vi "Main.vi"() -> ()   [LabVIEW 2012]
uses:
  UIAction.ctl
  UIActionQueueElement.ctl
  HeaterAction.ctl
  HeaterActionQueueElement.ctl
  MFCAction.ctl
  MFCActionQueueElement.ctl
  libs/LV-Utilities/LV-Utilities.lvlib
  LogAction.ctl
  LogActionQueueElement.ctl
  <vilib>/Utility/error.llb/DialogType.ctl
  HardwareAction.ctl
  HardwareActionQueueElement.ctl
  HeaterConfigurationGlobalAction.ctl
  MFCConfigurationGlobalAction.ctl
panel:
  in  "Chamber":u16(ring) items=["Chamber Name"]
  in  "NEXT CHAMBER":bool
  in  "PREVIOUS CHAMBER":bool
  in  "REMOVE CHAMBER":bool
  in  "ADD CHAMBER":bool
  out "MFC COM Port":u8=1
  out "Heater COM Port":u8=1
  in  "CONFIGURE HEATER":bool
  in  "PLOT MFC":bool
  in  "PLOT HEATER":bool
  in  "LOG START":bool
  out "Log Running?":bool
  in  "RESET":bool
  in  "SAVE":bool
  in  "OPEN":bool
  out "MFC Serial Number":string="Serial Number"
  in  "SELECT CONFIG":bool
  out "Setup File":path
  in  "CONFIGURE MFC":bool
  out "Heater Actual Slide":dbl(slide) scale=0.0..200.0 scale format="%#.1f"
  out "Heater Actual (C)":dbl=nan format="%.1f"
  out "Heater Setpoint Slide":dbl(slide) scale=0.0..200.0 scale format="%#.1f"
  out "Heater Setpoint (C)":dbl=nan format="%.1f"
  out "Heater State":enum16{"Not Connected", "Run", "Standby"}(ring)
  out "MFC Actual Slide":dbl(slide) scale=0.0..1000.0 scale format="%#.1f"
  out "MFC Actual (mL/min)":dbl=nan format="%.1f"
  out "MFC Setpoint Slide":dbl(slide) scale=0.0..1000.0 scale format="%#.1f"
  out "MFC Setpoint (mL/min)":dbl=nan format="%.1f"
  out "MFC Valve State":T1(ring)
  in  "DONE":bool
  # "Vacuum Pump"
  # "COM Port:"
  # "COM Port:"
  # "LOG"
  # "SETUP"
  # "Config File:"
  # "Actual"
  # "Setpoint"
  # "Actual"
  # "Setpoint"
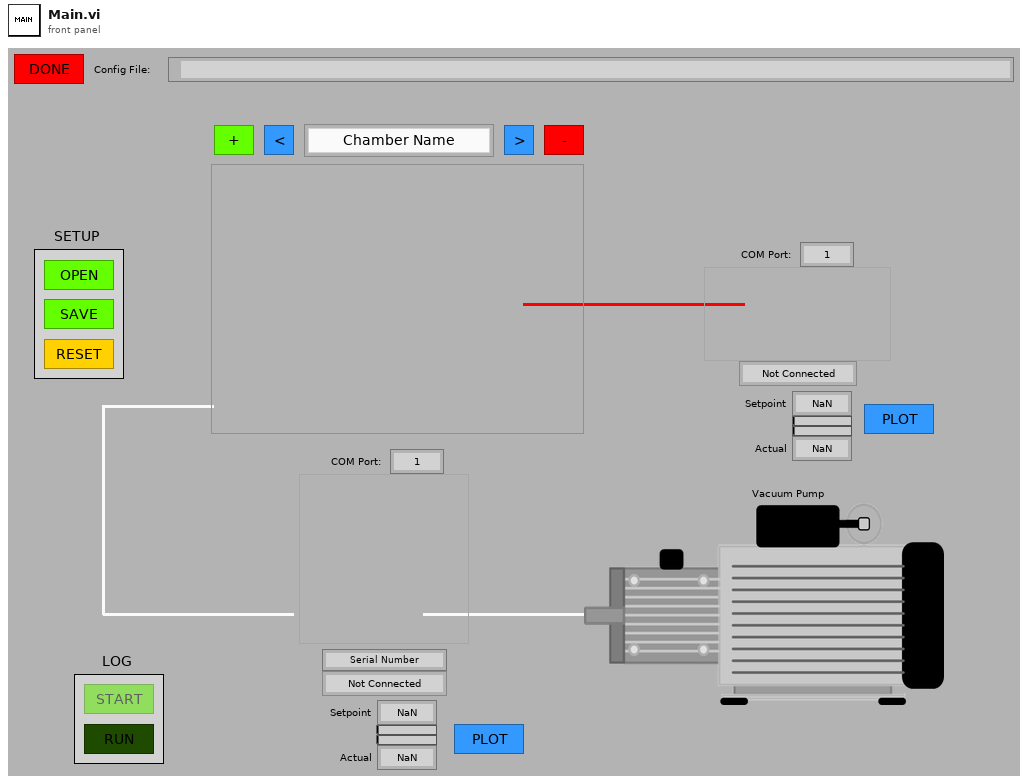
[diagram p1: front panel]
types:
  T1 = enum16{"Not Connected", "Automatic", "Closed", "Purge"}
  T2 = typedef "DataStructures.ctl" = cluster{"Display":refnum<notifier>, "Log":refnum<queue>}
  T3 = typedef "ActionQueues.ctl" = cluster{"UI Action":refnum<queue>, "Hardware Action":refnum<queue>, "Heater Action":refnum<queue>, "MFC Action":refnum<queue>, "Log Action":refnum<queue>}
  T4 = typedef "ExecutableConfiguration.ctl" = cluster{"Default Chamber Folder Path":path, "Default Log Folder Path":path, "Default Monitor":i32, "Center on Monitor?":bool}
  T5 = typedef "MFCActionQueueElement.ctl" = cluster{"Action":T6, "Data":variant}
  T6 = typedef "MFCAction.ctl" = enum16{"Initialize", "Start", "Read", "Write", "Stop", "Error", "Shutdown"}
  T7 = typedef "HeaterActionQueueElement.ctl" = cluster{"Action":T8, "Data":variant}
  T8 = typedef "HeaterAction.ctl" = enum16{"Initialize", "Start", "Read", "Write", "Stop", "Error", "Shutdown"}
  T9 = typedef "HardwareActionQueueElement.ctl" = cluster{"Action":T10, "Data":variant}
  T10 = typedef "HardwareAction.ctl" = enum16{"Initialize", "Collect", "Shutdown"}
  T11 = typedef "LogActionQueueElement.ctl" = cluster{"Action":T12, "Data":variant}
  T12 = typedef "LogAction.ctl" = enum16{"Initialize", "Start", "Log", "Stop", "Error", "Shutdown"}
  T13 = typedef "MFCConfigurationGlobalAction.ctl" = enum16{"Init", "Get", "Set", "Add", "Remove", "Reset"}
  T14 = typedef "HeaterConfigurationGlobalAction.ctl" = enum16{"Init", "Get", "Set", "Add", "Remove", "Reset"}
  T15 = enum8{"Enabled", "Disabled", "Disabled and Grayed Out"}
  T16 = typedef "UIActionQueueElement.ctl" = cluster{"Action":T17, "Data":variant}
  T17 = typedef "UIAction.ctl" = enum16{"Initialize", "Connect", "MFC Connected", "Heater Connected", "Disconnect", "MFC Disconnected", "Heater Disconnected", "Configure MFC", "Configure Heater", "Open Log", "Close Log", "Shutdown"}
  T18 = typedef "Setup.ctl" = cluster{"Chamber Name":string, "Log Folder Path":path, "Heater":T19, "MFC":T20}
  T19 = typedef "HeaterConfiguration.ctl" = cluster{"COM Port":u8, "Setpoint":dbl, "Standby?":bool}
  T20 = typedef "MFCConfiguration.ctl" = cluster{"COM Port":u32, "Timeout (msec)":u32, "Setpoint":dbl, "Valve State":T21, "Gas":T22, "Units":T23, "Serial Number":string, "Firmware Version":string}
  T21 = typedef "Sierra-M100.lvlib/ValveState.ctl" = enum16{"Automatic", "Closed", "Purge"}
  T22 = typedef "Sierra-M100.lvlib/Gas.ctl" = enum16{"Air", "Argon", "CO2", "CO", "Helium", "Hydrogen", "Methane", "Nitrogen", "Nitrous Oxide", "Oxygen"}
  T23 = typedef "Sierra-M100.lvlib/Units.ctl" = enum16{"scc/s", "scc/m", "scc/H", "Ncc/s", "Ncc/m", "Ncc/H", "SCF/s", "SCF/m", "SCF/H", "NM3/s", "NM3/m", "NM3/H", "SM3/s", "SM3/m", "SM3/H", "sl/s", "sl/m", "sl/H", "NL/s", "NL/m", "Nl/H", "g/s", "g/m", "g/H", "kg/s", "kg/m", "kg/H", "lb/s", "lb/m", "lb/H"}
  T24 = cluster{"Setpoint (mL/min)":dbl, "Actual (mL/min)":dbl}[]
  T25 = cluster{"Setpoint (mL/min)":dbl, "Actual (mL/min)":dbl}
  T26 = typedef "DialogType.ctl" = u16
  T27 = typedef "HardwareDisplayData.ctl" = cluster{"Heater":dbl, "MFC":dbl}
  T28 = typedef "MFCDisplayValveState.ctl" = enum16{"Not Connected", "Automatic", "Closed", "Purge"}
  T29 = typedef "HeaterDisplayState.ctl" = enum16{"Not Connected", "Run", "Standby"}
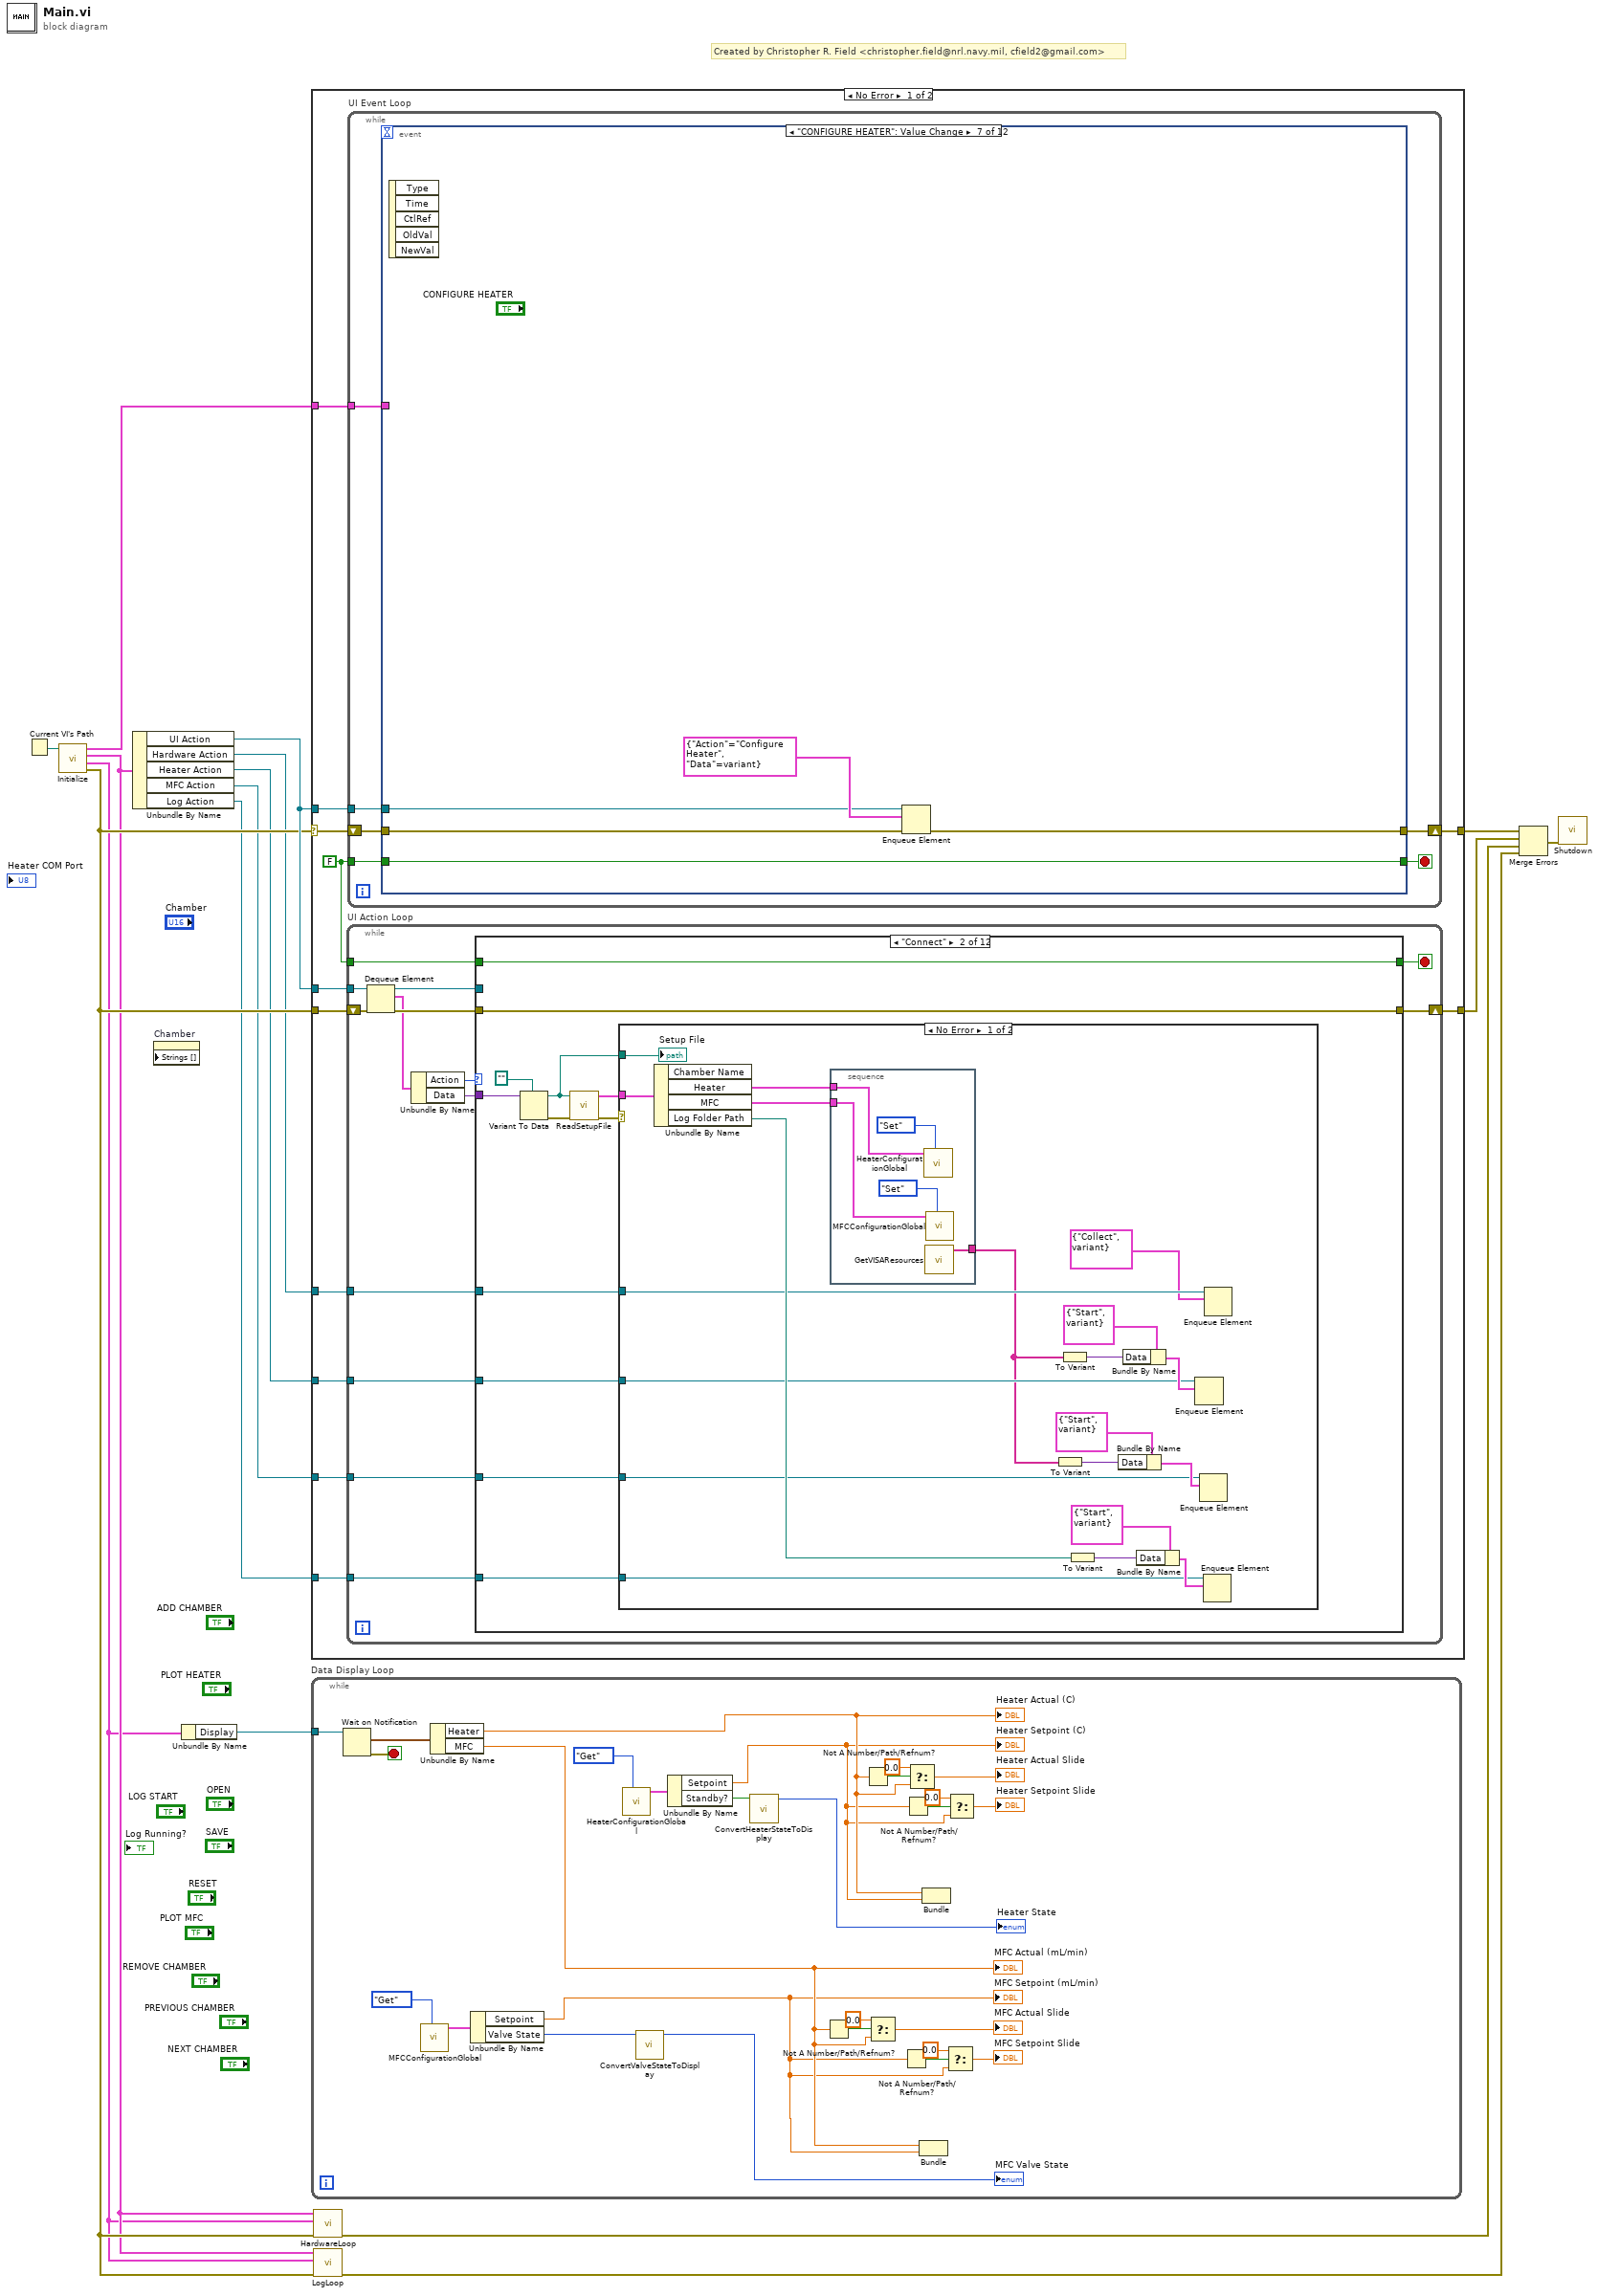
[diagram p0: block diagram]
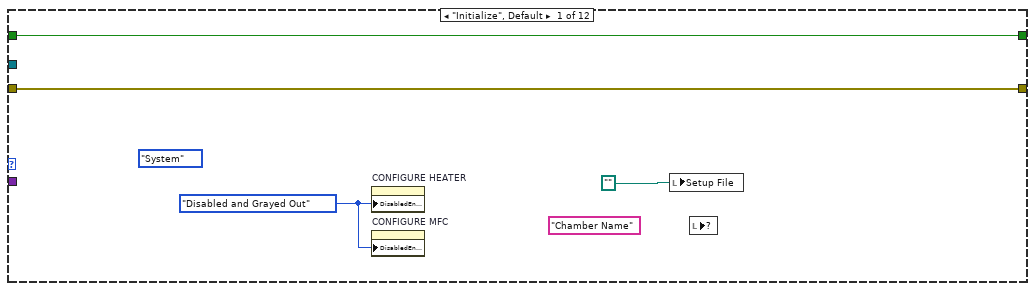
[diagram p2: hidden frame]
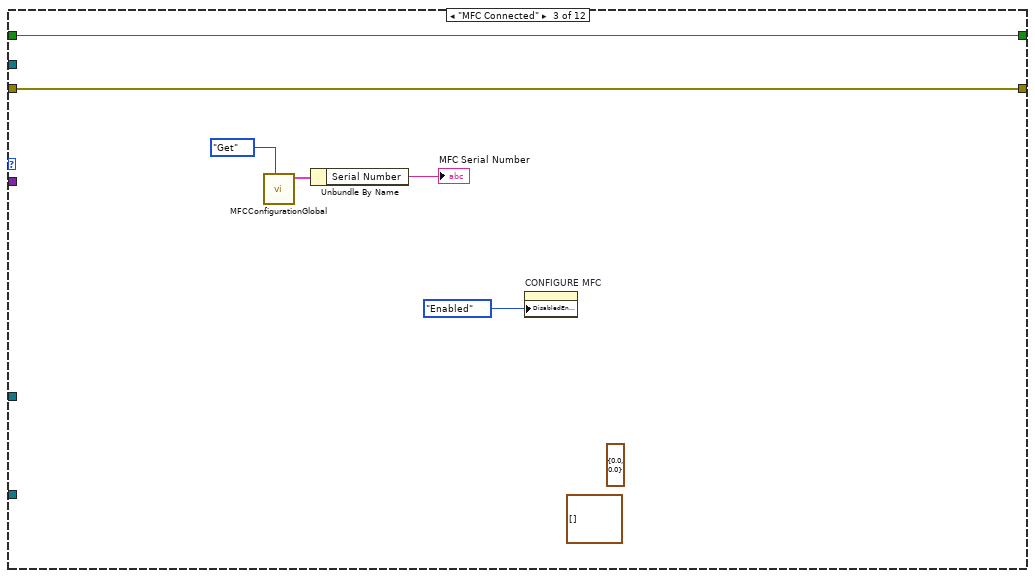
[diagram p4: hidden frame]
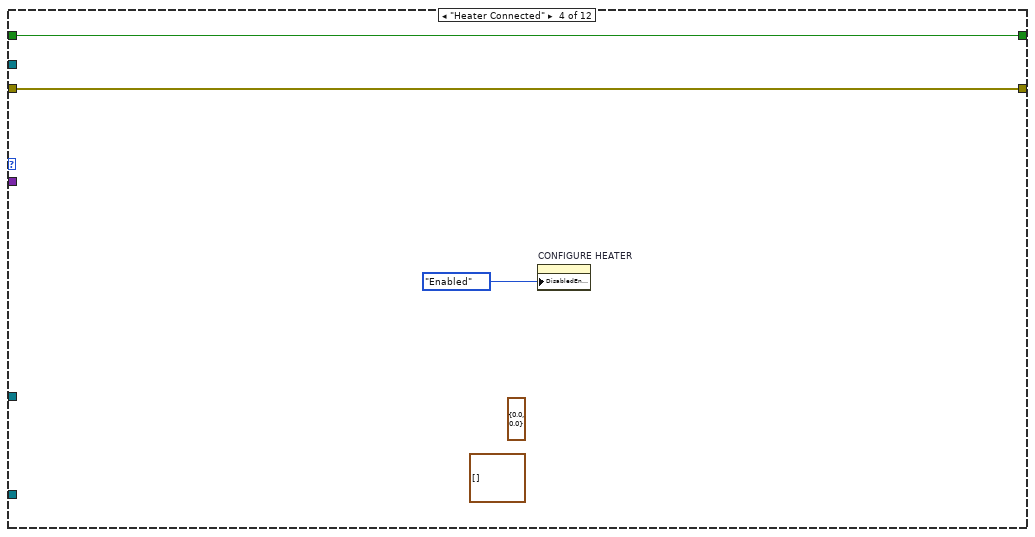
[diagram p5: hidden frame]
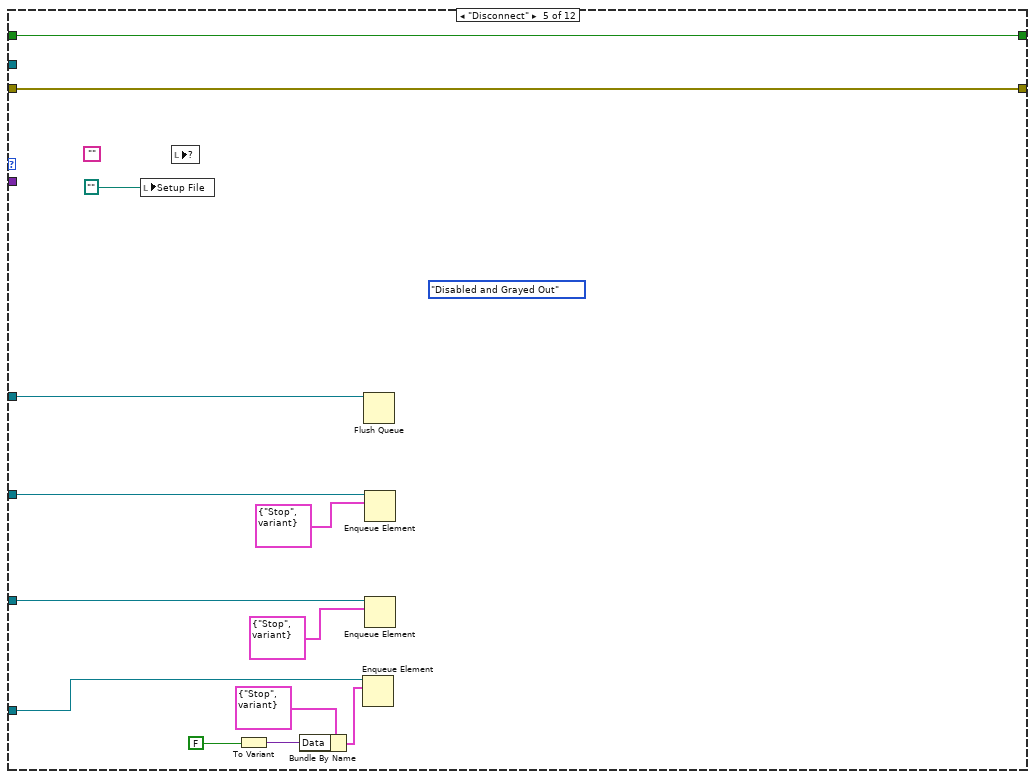
[diagram p6: hidden frame]
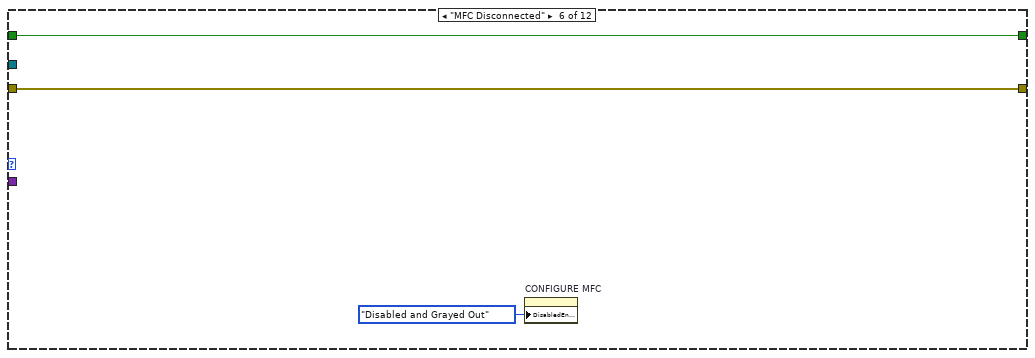
[diagram p7: hidden frame]
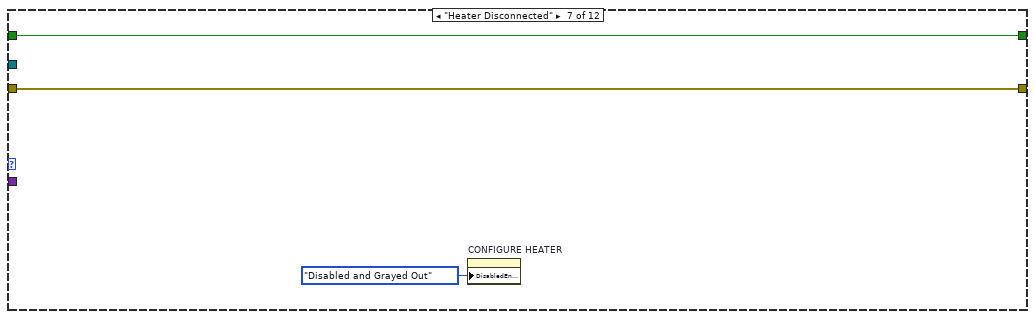
[diagram p8: hidden frame]
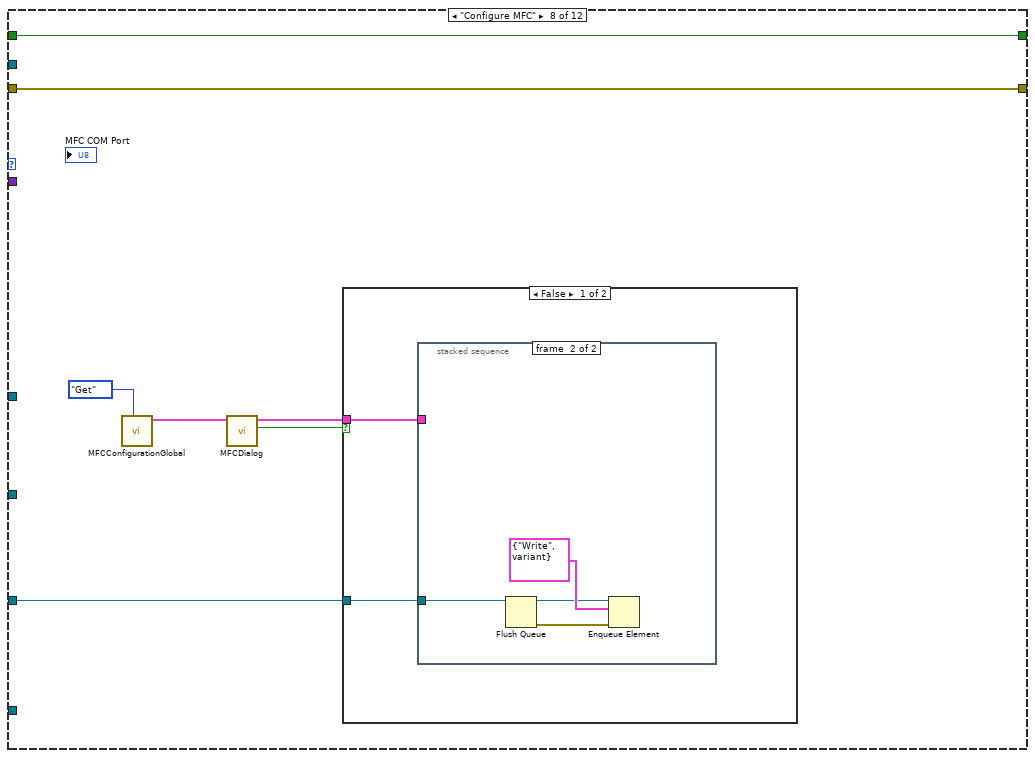
[diagram p9: hidden frame]
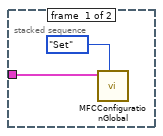
[diagram p10: hidden frame]
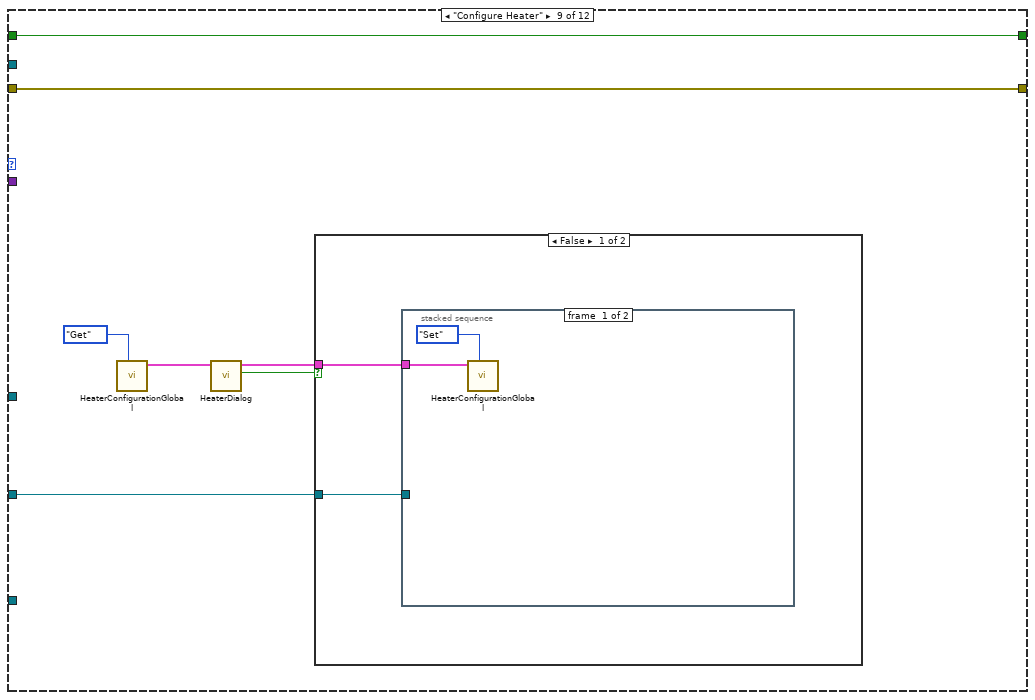
[diagram p12: hidden frame]
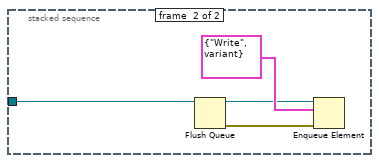
[diagram p13: hidden frame]
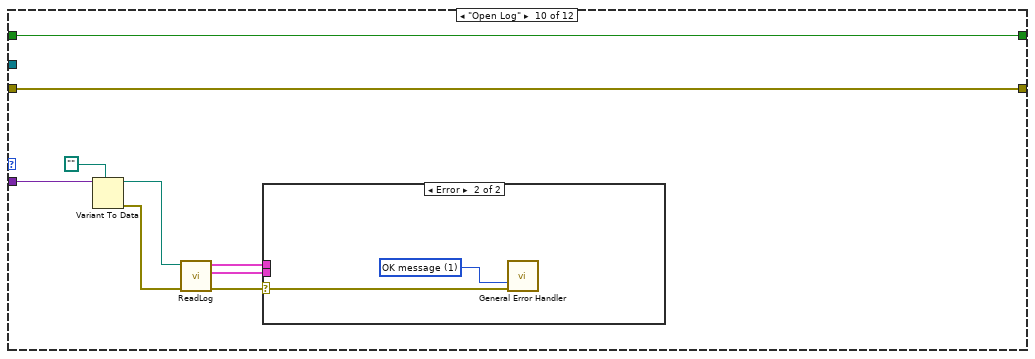
[diagram p15: hidden frame]
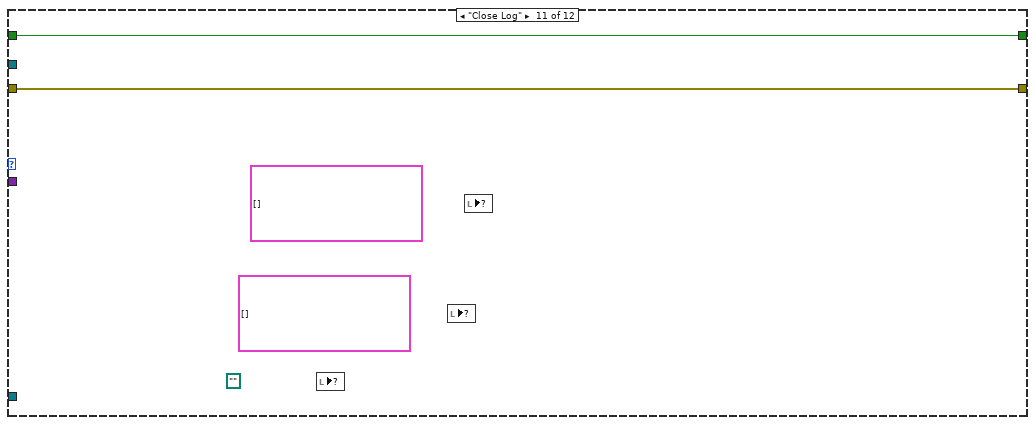
[diagram p17: hidden frame]
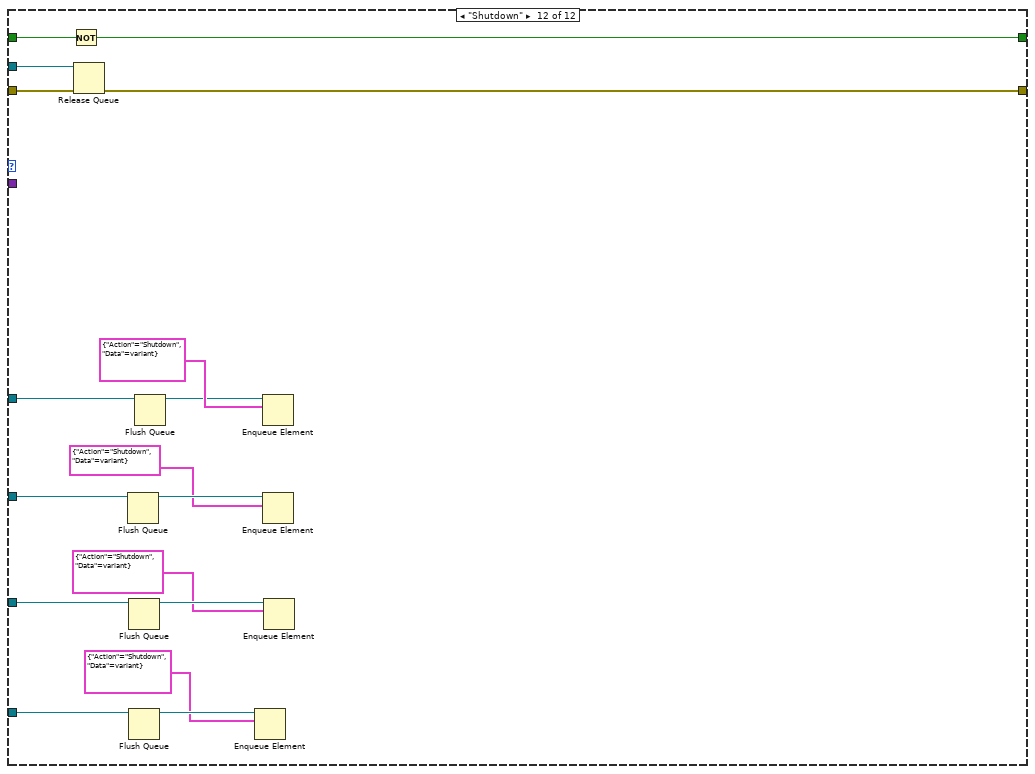
[diagram p18: hidden frame]
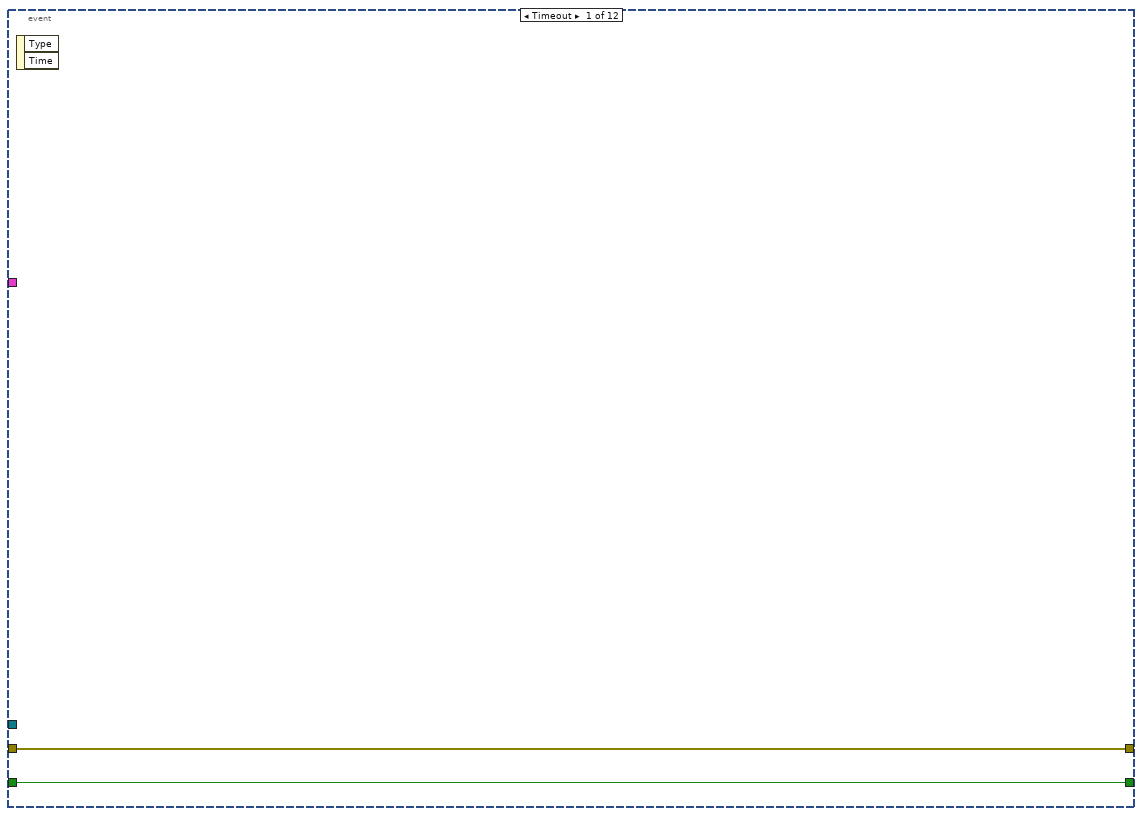
[diagram p19: hidden frame]
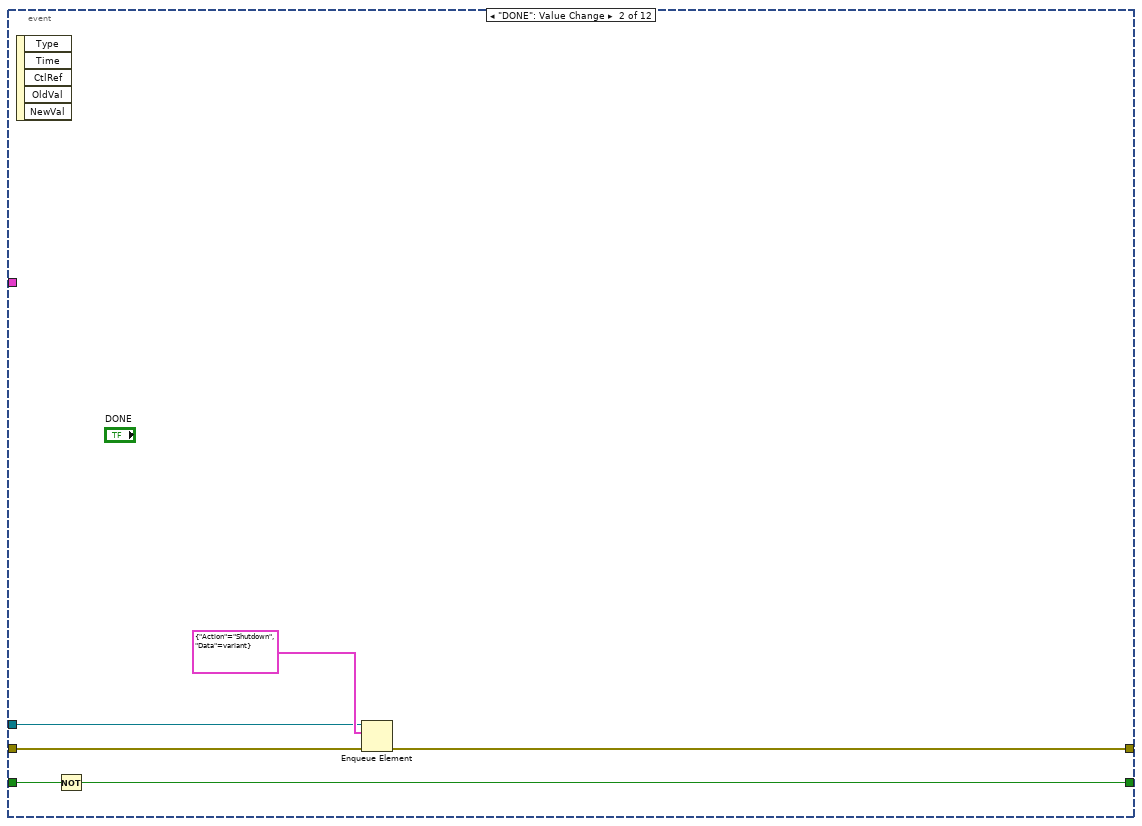
[diagram p20: hidden frame]
diagram:
  # "Created by Christopher R. Field <christopher.field@nrl.navy.mil, cfield2@gmail.com>"
  n1 = Current VI's Path() -> (path=w16:path)
  n2 = call "Initialize.vi"("VI Path"=w16) -> ("Error Out"=w11:errorcluster, "Data Structures"=w6:T2, "Action Queues"=w7:T3, "Executable Configuration"=w4:T4)  [unwired: 7 in]
  n3 = Unbundle By Name(w7) -> ("UI Action"=w15:refnum<queue>, "Hardware Action"=w8:refnum<queue>, "Heater Action"=w3:refnum<queue>, "MFC Action"=w2:refnum<queue>, "Log Action"=w1:refnum<queue>)
  n4 = property on="Chamber" class="Ring (strict)" props=["Strings []"]() -> ()  [unwired: 3 in, 2 out]
  n5 = Unbundle By Name(w6) -> ("Display"=w5:refnum<notifier>)
  n6 = case shown="No Error" w11 {
    selector: w11 -> [w27 w255]
    tunnel: [w28 w255] -> w14
    tunnel: w15 -> [w25 _]
    tunnel: w11 -> [w24 w254]
    tunnel: w15 -> [w23 _]
    tunnel: [w22 w254] -> w13
    tunnel: w8 -> [w21 _]
    tunnel: w4 -> [w20 _]
    tunnel: w3 -> [w19 _]
    tunnel: w2 -> [w18 _]
    tunnel: w1 -> [w17 _]
    frame No Error {
      w26 = FALSE
      n7 = while "UI Action Loop" {
        tunnel: w26 -> [w42]
        tunnel: w25 -> [w32]
        shift-right: [w35] -> w22
        shift-left: w24 -> [w41]
        tunnel: w21 -> [w33]
        tunnel: w19 -> [w31]
        tunnel: w18 -> [w30]
        tunnel: w17 -> [w29]
        stop <- w34 stop-if-true
        n8 = Dequeue Element(queue=w32, error in (no error)=w41) -> (queue out=w40:refnum<queue>, element=w38:T16, error out=w39:errorcluster)  [unwired: 1 in, 1 out]
        n9 = Unbundle By Name(w38) -> ("Action"=w37:T17, "Data"=w36:variant)
        n10 = case shown="\"Connect\"" w37 {
          tunnel: w42 -> [w46 w58 w89 w91 w105 w108 w111 w118 w133 w150 w154 w171]
          tunnel: w40 -> [_ _ _ _ _ _ _ _ _ _ _ w169]
          tunnel: w39 -> [w45 w57 w88 w92 w104 w107 w110 w117 w132 w149 w153 w168]
          tunnel: w36 -> [_ w56 _ _ _ _ _ _ _ w148 _ _]
          tunnel: [w45 w57 w88 w92 w104 w107 w110 w117 w132 w149 w153 w167] -> w35
          tunnel: [w46 w58 w89 w91 w105 w108 w111 w118 w133 w150 w154 w170] -> w34
          tunnel: w33 -> [_ w50 _ _ w93 _ _ _ _ _ _ w156]
          tunnel: w31 -> [_ w49 _ _ w96 _ _ _ w131 _ _ w160]
          tunnel: w30 -> [_ w48 _ _ w95 _ _ w116 _ _ _ w159]
          tunnel: w29 -> [_ w47 _ _ w94 _ _ _ _ _ _ w158]
          frame "Initialize", Default {
            (unwired) "Chamber Name" ("Chamber Name")
            w44 = T15."Disabled and Grayed Out" ("Disabled")
            (unwired) enum32{"System", "Live", "Logs"}."System" ("Tab Control")
            n11 = property on="CONFIGURE HEATER" class="Bool"("DisabledEnum"=w44) -> ()  [unwired: 2 in, 2 out]
            n12 = property on="CONFIGURE MFC" class="Bool"("DisabledEnum"=w44) -> ()  [unwired: 2 in, 2 out]
            n13 = local write "Setup File"(path "") -> ()
            n14 = local read item#-1() -> ()  [unwired: 1 in]
          }
          frame "Connect" {
            n15 = Variant To Data(type=path "", Variant=w56) -> (data=w51:path, error out=w54:errorcluster)  [unwired: 1 in]
            n16 = call "ReadSetupFile.vi"("Error In"=w54, "Setup File"=w51) -> ("Error Out"=w53:errorcluster, "Setup"=w52:T18)  [unwired: 8 in]
            n17 = case shown="No Error" w53 {
              tunnel: w52 -> [w78 _]
              tunnel: w51 -> [w77 _]
              tunnel: w50 -> [w72 _]
              tunnel: w49 -> [w65 _]
              tunnel: w48 -> [w64 _]
              tunnel: w47 -> [w62 _]
              frame No Error {
                n18 = Unbundle By Name(w78) -> ("Heater"=w61:T19, "MFC"=w60:T20, "Log Folder Path"=w74:path)  [unwired: 1 out]
                n19 = stacked-sequence {
                  tunnel: w61 -> [w82]
                  tunnel: w60 -> [w81]
                  tunnel: [w79] -> w59
                  frame #0 {
                    n20 = call "HeaterConfigurationGlobal.vi"("Action"=HeaterConfigurationGlobalAction."Set", "Set Value"=w82) -> ()  [unwired: 9 in, 1 out]
                    n21 = call "GetVISAResources.vi"() -> ("VISA Resources"=w79:string[])  [unwired: 10 in, 1 out]
                    n22 = call "MFCConfigurationGlobal.vi"("Action"=MFCConfigurationGlobalAction."Set", "Set Value"=w81) -> ()  [unwired: 9 in, 1 out]
                  }
                }
                n23 = To Variant(anything=w59) -> (Variant=w68:variant)
                n24 = To Variant(anything=w59) -> (Variant=w70:variant)
                n25 = To Variant(anything=w74) -> (Variant=w75:variant)
                n26 = Bundle By Name(cluster=T5 {"Action"=enum."Start", "Data"=variant} ("element"), "Data"=w68) -> (w66:T5)
                n27 = Bundle By Name(cluster=T7 {"Action"=enum."Start", "Data"=variant} ("element"), "Data"=w70) -> (w69:T7)
                n28 = Bundle By Name(cluster=T11 {"Action"=enum."Start", "Data"=variant} ("element"), "Data"=w75) -> (w73:T11)
                n29 = Enqueue Element(queue=w65, element=w69) -> ()  [unwired: 2 in, 3 out]
                n30 = Enqueue Element(queue=w64, element=w66) -> ()  [unwired: 2 in, 3 out]
                n31 = Enqueue Element(queue=w62, element=w73) -> ()  [unwired: 2 in, 3 out]
                n32 = Enqueue Element(queue=w72, element=T9 {"Action"=enum."Collect", "Data"=variant}) -> ()  [unwired: 2 in, 3 out]
                "Setup File" <- w77
              }
              frame Error {
              }
            }
          }
          frame "MFC Connected" {
            (unwired) T24 [] ("History Data")
            (unwired) T25 {"Setpoint (mL/min)"=0.0, "Actual (mL/min)"=0.0} ("Live MFC Chart")
            n33 = call "MFCConfigurationGlobal.vi"("Action"=MFCConfigurationGlobalAction."Get") -> ("Value Out"=w85:T20)  [unwired: 10 in]
            n34 = Unbundle By Name(w85) -> ("Serial Number"=→"MFC Serial Number":string)
            n35 = property on="CONFIGURE MFC" class="Bool"("DisabledEnum"=T15."Enabled" ("Disabled")) -> ()  [unwired: 2 in, 2 out]
          }
          frame "Heater Connected" {
            (unwired) cluster{"Setpoint (C)":dbl, "Actual (C)":dbl}[] [] ("History Data")
            (unwired) cluster{"Setpoint (C)":dbl, "Actual (C)":dbl} {"Setpoint (C)"=0.0, "Actual (C)"=0.0} ("Live Heater Chart")
            n36 = property on="CONFIGURE HEATER" class="Bool"("DisabledEnum"=T15."Enabled" ("Disabled")) -> ()  [unwired: 2 in, 2 out]
          }
          frame "Disconnect" {
            (unwired) T15."Disabled and Grayed Out" ("Disabled")
            (unwired) ""
            n37 = local write "Setup File"(path "") -> ()
            n38 = local read item#-1() -> ()  [unwired: 1 in]
            n39 = To Variant(anything=FALSE) -> (Variant=w99:variant)
            n40 = Bundle By Name(cluster=T11 {"Action"=enum."Stop", "Data"=variant} ("element"), "Data"=w99) -> (w97:T11)
            n41 = Enqueue Element(queue=w94, element=w97) -> ()  [unwired: 2 in, 3 out]
            n42 = Flush Queue(queue=w93) -> ()  [unwired: 1 in, 3 out]
            n43 = Enqueue Element(queue=w96, element=T7 {"Action"=enum."Stop", "Data"=variant}) -> ()  [unwired: 2 in, 3 out]
            n44 = Enqueue Element(queue=w95, element=T5 {"Action"=enum."Stop", "Data"=variant}) -> ()  [unwired: 2 in, 3 out]
          }
          frame "MFC Disconnected" {
            n45 = property on="CONFIGURE MFC" class="Bool"("DisabledEnum"=T15."Disabled and Grayed Out" ("Disabled")) -> ()  [unwired: 2 in, 2 out]
          }
          frame "Heater Disconnected" {
            n46 = property on="CONFIGURE HEATER" class="Bool"("DisabledEnum"=T15."Disabled and Grayed Out" ("Disabled")) -> ()  [unwired: 2 in, 2 out]
          }
          frame "Configure MFC" {
            n47 = call "MFCConfigurationGlobal.vi"("Action"=MFCConfigurationGlobalAction."Get") -> ("Value Out"=w114:T20)  [unwired: 10 in]
            n48 = call "MFCDialog.vi"("MFC Configuration In"=w114) -> ("Cancelled?"=w113:bool, "MFC Configuration Out"=w112:T20)  [unwired: 8 in, 1 out]
            n49 = case shown="False" w113 {
              tunnel: w116 -> [w120 _]
              tunnel: w112 -> [w119 _]
              frame False {
                n50 = stacked-sequence {
                  tunnel: w120 -> [_ w123]
                  tunnel: w119 -> [w122 _]
                  frame #0 {
                    n51 = call "MFCConfigurationGlobal.vi"("Action"=MFCConfigurationGlobalAction."Set", "Set Value"=w122) -> ()  [unwired: 9 in, 1 out]
                  }
                  frame #1 {
                    n52 = Flush Queue(queue=w123) -> (queue out=w125:refnum<queue>, error out=w124:errorcluster)  [unwired: 1 in, 1 out]
                    n53 = Enqueue Element(queue=w125, element=T5 {"Action"=enum."Write", "Data"=variant}, error in (no error)=w124) -> ()  [unwired: 1 in, 3 out]
                  }
                }
              }
              frame True {
              }
            }
          }
          frame "Configure Heater" {
            n54 = call "HeaterConfigurationGlobal.vi"("Action"=HeaterConfigurationGlobalAction."Get") -> ("Value Out"=w129:T19)  [unwired: 10 in]
            n55 = call "HeaterDialog.vi"("Heater Configuration In"=w129) -> ("Cancelled?"=w128:bool, "Heater Configuration Out"=w127:T19)  [unwired: 8 in, 1 out]
            n56 = case shown="False" w128 {
              tunnel: w131 -> [w135 _]
              tunnel: w127 -> [w134 _]
              frame False {
                n57 = stacked-sequence {
                  tunnel: w135 -> [_ w138]
                  tunnel: w134 -> [w137 _]
                  frame #0 {
                    n58 = call "HeaterConfigurationGlobal.vi"("Action"=HeaterConfigurationGlobalAction."Set", "Set Value"=w137) -> ()  [unwired: 9 in, 1 out]
                  }
                  frame #1 {
                    n59 = Flush Queue(queue=w138) -> (queue out=w140:refnum<queue>, error out=w139:errorcluster)  [unwired: 1 in, 1 out]
                    n60 = Enqueue Element(queue=w140, element=T7 {"Action"=enum."Write", "Data"=variant}, error in (no error)=w139) -> ()  [unwired: 1 in, 3 out]
                  }
                }
              }
              frame True {
              }
            }
          }
          frame "Open Log" {
            n61 = Variant To Data(type=path "", Variant=w148) -> (data=w146:path, error out=w142:errorcluster)  [unwired: 1 in]
            n62 = call "ReadLog.vi"("Error In"=w142, "Log File Path"=w146) -> ("Error Out"=w145:errorcluster, "MFC Plots"=w143:cluster{timestamp[], "Y Data":dbl[]}[], "Heater Plots"=w144:cluster{timestamp[], "Y Data":dbl[]}[])  [unwired: 7 in]
            n63 = case shown="Error" w145 {
              selector: w145 -> [_ w152]
              tunnel: w144 -> [_ _]
              tunnel: w143 -> [_ _]
              frame No Error {
              }
              frame Error {
                w151 = T26 1 items=["no dialog", "OK message", "continue or stop message", "OK message + warnings", "continue/stop + warnings"] ("type of dialog (OK msg:1)")
                n64 = call <vilib>:"General Error Handler.vi"("type of dialog (OK msg:1)"=w151, "error in (no error)"=w152) -> ()  [unwired: 9 in, 5 out]
              }
            }
          }
          frame "Close Log" {
            (unwired) path ""
            (unwired) cluster{timestamp[], "Y Data":dbl[]}[] [] ("MFC Graph")
            (unwired) cluster{timestamp[], "Y Data":dbl[]}[] [] ("Heater Graph")
            n65 = local read item#-1() -> ()  [unwired: 1 in]
            n66 = local read item#-1() -> ()  [unwired: 1 in]
            n67 = local read item#-1() -> ()  [unwired: 1 in]
          }
          frame "Shutdown" {
            n68 = Not(x=w171) -> (.not. x?=w170:bool)
            n69 = Release Queue(queue=w169, error in (no error)=w168) -> (error out=w167:errorcluster)  [unwired: 1 in, 2 out]
            n70 = Flush Queue(queue=w160) -> (queue out=w166:refnum<queue>)  [unwired: 1 in, 2 out]
            n71 = Flush Queue(queue=w159) -> (queue out=w164:refnum<queue>)  [unwired: 1 in, 2 out]
            n72 = Flush Queue(queue=w158) -> (queue out=w162:refnum<queue>)  [unwired: 1 in, 2 out]
            n73 = Flush Queue(queue=w156) -> (queue out=w155:refnum<queue>)  [unwired: 1 in, 2 out]
            n74 = Enqueue Element(queue=w162, element=T11 {"Action"=enum."Shutdown", "Data"=variant}) -> ()  [unwired: 2 in, 3 out]
            n75 = Enqueue Element(queue=w155, element=T9 {"Action"=enum."Shutdown", "Data"=variant}) -> ()  [unwired: 2 in, 3 out]
            n76 = Enqueue Element(queue=w166, element=T7 {"Action"=enum."Shutdown", "Data"=variant}) -> ()  [unwired: 2 in, 3 out]
            n77 = Enqueue Element(queue=w164, element=T5 {"Action"=enum."Shutdown", "Data"=variant}) -> ()  [unwired: 2 in, 3 out]
          }
        }
      }
      n78 = while "UI Event Loop" {
        tunnel: w26 -> [w177]
        shift-right: [w174] -> w28
        shift-left: w27 -> [w175]
        tunnel: w23 -> [w173]
        tunnel: w20 -> [w172]
        stop <- w176 stop-if-true
        n79 = event shown="[6] \"CONFIGURE HEATER\": Value Change" {
          selector: _ -> [_ _ _ _ _ _ _ _ _ _ _ _]
          dyn-events: _ -> [_ _ _ _ _ _ _ _ _ _ _ _]
          timeout: _ -> [_ _ _ _ _ _ _ _ _ _ _ _]
          tunnel: w177 -> [w179 w185 w191 w193 w195 w197 w202 w207 w209 w219 w240 w253]
          tunnel: [w179 w184 w190 w193 w195 w197 w202 w207 w209 w219 w240 w253] -> w176
          tunnel: w175 -> [w178 w183 w188 w192 w194 w196 w201 w206 w208 w214 w234 w252]
          tunnel: [w178 w182 w187 w192 w194 w196 w200 w205 w208 w213 w233 w251] -> w174
          tunnel: w173 -> [_ w180 w186 _ _ _ w198 w203 _ w215 w235 w249]
          tunnel: w172 -> [_ _ _ _ _ _ _ _ _ w210 w231 _]
          event Timeout {
            n80 = event-data() -> ()  [unwired: 1 in, 2 out]
          }
          event "DONE": Value Change {
            n81 = event-data() -> ()  [unwired: 1 in, 5 out]
            n82 = Not(x=w185) -> (.not. x?=w184:bool)
            n83 = Enqueue Element(queue=w180, element=T16 {"Action"=enum."Shutdown", "Data"=variant}, error in (no error)=w183) -> (error out=w182:errorcluster)  [unwired: 1 in, 2 out]
          }
          event Panel Close? {
            n84 = event-data() -> ()  [unwired: 1 in, 3 out]
            n85 = Not(x=w191) -> (.not. x?=w190:bool)
            n86 = Enqueue Element(queue=w186, element=T16 {"Action"=enum."Shutdown", "Data"=variant}, error in (no error)=w188) -> (error out=w187:errorcluster)  [unwired: 1 in, 2 out]
            n87 = event-data("Discard?"=w190) -> ()  [unwired: 1 in, 1 out]
          }
          event #3 (no event record) {
            (unwired) enum32{"System", "Live", "Logs"}."System" ("Tab Control")
            n88 = event-data() -> ()  [unwired: 1 in, 5 out]
          }
          event #4 (no event record) {
            (unwired) enum32{"System", "Live", "Logs"}."Live" ("Tab Control")
            n89 = event-data() -> ()  [unwired: 1 in, 5 out]
          }
          event #5 (no event record) {
            (unwired) enum32{"System", "Live", "Logs"}."Logs" ("Tab Control")
            n90 = event-data() -> ()  [unwired: 1 in, 5 out]
          }
          event "CONFIGURE HEATER": Value Change {
            n91 = event-data() -> ()  [unwired: 1 in, 5 out]
            n92 = Enqueue Element(queue=w198, element=T16 {"Action"=enum."Configure Heater", "Data"=variant}, error in (no error)=w201) -> (error out=w200:errorcluster)  [unwired: 1 in, 2 out]
          }
          event "CONFIGURE MFC": Value Change {
            n93 = event-data() -> ()  [unwired: 1 in, 5 out]
            n94 = Enqueue Element(queue=w203, element=T16 {"Action"=enum."Configure MFC", "Data"=variant}, error in (no error)=w206) -> (error out=w205:errorcluster)  [unwired: 1 in, 2 out]
          }
          event #8 (no event record) {
            (unwired) T24 [] ("History Data")
            (unwired) T25 {"Setpoint (mL/min)"=0.0, "Actual (mL/min)"=0.0} ("Live MFC Chart")
            (unwired) cluster{"Setpoint (C)":dbl, "Actual (C)":dbl}[] [] ("History Data")
            (unwired) cluster{"Setpoint (C)":dbl, "Actual (C)":dbl} {"Setpoint (C)"=0.0, "Actual (C)"=0.0} ("Live Heater Chart")
            n95 = event-data() -> ()  [unwired: 1 in, 5 out]
          }
          event "SELECT CONFIG": Value Change {
            n96 = event-data() -> ()  [unwired: 1 in, 5 out]
            n97 = Unbundle By Name(w210) -> ("Default Chamber Folder Path"=w211:path)
            n98 = call "SelectFile.vi"("File Description"="Chamber Configuration File", "File Extension (.*)"=".ini", "Start Path"=w211) -> ("Cancelled?"=w216:bool, "Selected File Path"=w212:path)  [unwired: 6 in, 1 out]
            n99 = case shown="False" w216 {
              tunnel: w215 -> [w220 _]
              tunnel: w214 -> [w224 w230]
              tunnel: [w229 w230] -> w213
              tunnel: w212 -> [w226 _]
              frame False {
                n100 = To Variant(anything=w226) -> (Variant=w227:variant)
                n101 = Bundle By Name(cluster=T16 {"Action"=enum."Connect", "Data"=variant} ("element"), "Data"=w227) -> (w225:T16)
                n102 = Enqueue Element(queue=w220, element=T16 {"Action"=enum."Disconnect", "Data"=variant}, error in (no error)=w224) -> (queue out=w222:refnum<queue>, error out=w223:errorcluster)  [unwired: 1 in, 1 out]
                n103 = Enqueue Element(queue=w222, element=w225, error in (no error)=w223) -> (error out=w229:errorcluster)  [unwired: 1 in, 2 out]
              }
              frame True {
              }
            }
          }
          event #10 (no event record) {
            n104 = event-data() -> ()  [unwired: 1 in, 5 out]
            n105 = Unbundle By Name(w231) -> ("Default Log Folder Path"=w232:path)
            n106 = call "SelectFile.vi"("File Description"="Sample Chamber Log File", "File Extension (.*)"=".log", "Start Path"=w232) -> ("Cancelled?"=w237:bool, "Selected File Path"=w236:path)  [unwired: 6 in, 1 out]
            n107 = case shown="False" w237 {
              tunnel: w236 -> [w242 _]
              tunnel: w235 -> [w241 _]
              tunnel: w234 -> [w247 w248]
              tunnel: [w246 w248] -> w233
              frame False {
                n108 = To Variant(anything=w242) -> (Variant=w243:variant)
                n109 = Bundle By Name(cluster=T16 {"Action"=enum."Open Log", "Data"=variant} ("element"), "Data"=w243) -> (w244:T16)
                n110 = Enqueue Element(queue=w241, element=w244, error in (no error)=w247) -> (error out=w246:errorcluster)  [unwired: 1 in, 2 out]
              }
              frame True {
              }
            }
          }
          event #11 (no event record) {
            n111 = event-data() -> ()  [unwired: 1 in, 5 out]
            n112 = Enqueue Element(queue=w249, element=T16 {"Action"=enum."Close Log", "Data"=variant}, error in (no error)=w252) -> (error out=w251:errorcluster)  [unwired: 1 in, 2 out]
          }
        }
      }
    }
    frame Error {
    }
  }
  n113 = while "Data Display Loop" {
    tunnel: w5 -> [w268]
    stop <- w282 stop-if-true
    n114 = Wait on Notification(notifier=w268) -> (notification=w269:T27, error out=w282:errorcluster)  [unwired: 3 in, 2 out]
    n115 = call "MFCConfigurationGlobal.vi"("Action"=MFCConfigurationGlobalAction."Get") -> ("Value Out"=w259:T20)  [unwired: 10 in]
    n116 = Unbundle By Name(w269) -> ("Heater"=w267:dbl, "MFC"=w266:dbl)
    "Heater Actual (C)" <- w267
    "MFC Actual (mL/min)" <- w266
    n117 = Unbundle By Name(w259) -> ("Setpoint"=w256:dbl, "Valve State"=w258:T21)
    "MFC Setpoint (mL/min)" <- w256
    n118 = call "HeaterConfigurationGlobal.vi"("Action"=HeaterConfigurationGlobalAction."Get") -> ("Value Out"=w264:T19)  [unwired: 10 in]
    n119 = call "ConvertValveStateToDisplay.vi"("Valve State"=w258) -> ("MFC Valve State"=→"MFC Valve State":T28)  [unwired: 10 in]
    n120 = Unbundle By Name(w264) -> ("Setpoint"=w263:dbl, "Standby?"=w262:bool)
    "Heater Setpoint (C)" <- w263
    n121 = call "ConvertHeaterStateToDisplay.vi"("Standby?"=w262) -> ("Heater Display State"=→"Heater State":T29)  [unwired: 10 in]
    n122 = Not A Number/Path/Refnum?(number/path/refnum=w266) -> (NaN/Path/Refnum?=w270:bool)
    n123 = Not A Number/Path/Refnum?(number/path/refnum=w267) -> (NaN/Path/Refnum?=w281:bool)
    n124 = Select(t=0.0, s=w270, f=w266) -> (s? t:f=→"MFC Actual Slide":dbl)
    n125 = Not A Number/Path/Refnum?(number/path/refnum=w256) -> (NaN/Path/Refnum?=w273:bool)
    n126 = Not A Number/Path/Refnum?(number/path/refnum=w263) -> (NaN/Path/Refnum?=w279:bool)
    n127 = Select(t=0.0, s=w281, f=w267) -> (s? t:f=→"Heater Actual Slide":dbl)
    n128 = Bundle("MFC"=w266, "Setpoint"=w256) -> ()  [unwired: 1 in, 1 out]
    n129 = Bundle("Heater"=w267, "Setpoint"=w263) -> ()  [unwired: 1 in, 1 out]
    n130 = Select(t=0.0, s=w273, f=w256) -> (s? t:f=→"MFC Setpoint Slide":dbl)
    n131 = Select(t=0.0, s=w279, f=w263) -> (s? t:f=→"Heater Setpoint Slide":dbl)
  }
  n132 = call "HardwareLoop.vi"("Error In"=w11, "Data Structures"=w6, "Action Queues"=w7) -> ("Error Out"=w10:errorcluster)  [unwired: 8 in]
  n133 = call "LogLoop.vi"("Error In"=w11, "Data Structures"=w6, "Action Queues"=w7) -> ("Error Out"=w9:errorcluster)  [unwired: 8 in]
  n134 = Merge Errors(w14, w13, w10, w9) -> (w12:errorcluster)
  n135 = call "Shutdown.vi"("Error In"=w12) -> ()  [unwired: 11 in]
